vi "Compute Max Level.vi"(0 "Tone in":refnum<class "Tone.lvclass">, 1 "Filter in":refnum<class "Filter.lvclass">, 5 "Level in":refnum<class "Level.lvclass">, 7 "Fs (Hz)":dbl, 9 "Vmax":dbl, 11 "error in (no error)":errorcluster) -> (4 "Tone out":refnum<class "Tone.lvclass">, 6 "Level out":refnum<class "Level.lvclass">, 10 "Lmax":dbl, 15 "error out":errorcluster)   [LabVIEW 2020, in "Tone.lvclass"]
uses:
  Tone.lvclass
  D:/Development/epl-vi-lib/Koop/KObject Class/KObject.lvclass
  Level/Level.lvclass
  Filter/Filter.lvclass
  Tone.lvclass/Tone.ctl
  Level/Level.lvclass/Level.ctl
  82eb419d-049d-446f-8907-0d6ace39b23e.vi
  24a302fd-cf4a-4809-a84c-42078eca26b2.vi
  e33db8c1-d80d-4f9e-86c8-a606ede5ff50.vi
  937cdd26-08b4-48c4-ab2b-7b4c98fffdd3.vi
  9062d80a-ea83-4365-b942-483c8a64e32a.vi
  Level/Read Units.vi
  Koop/KObject Class/KObject.lvclass
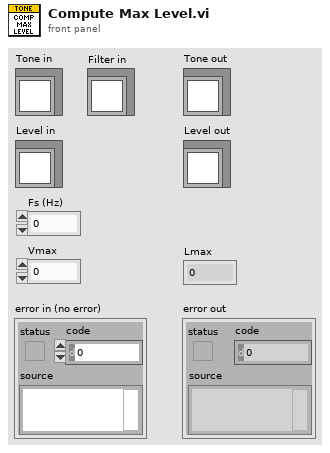
[diagram p1: front panel]
types:
  T1 = typedef "Level.lvclass/LevelUnits.ctl" = enum16{"dB atten", "dB SPL", "dB Vrms", "Volts", "dB mW", "mW", "dB HL", "dB SL"}
  T2 = cluster{"Freq (Hz)":dbl[], "Mag (dB SPL)":dbl[], "Phase (deg)":dbl[]}
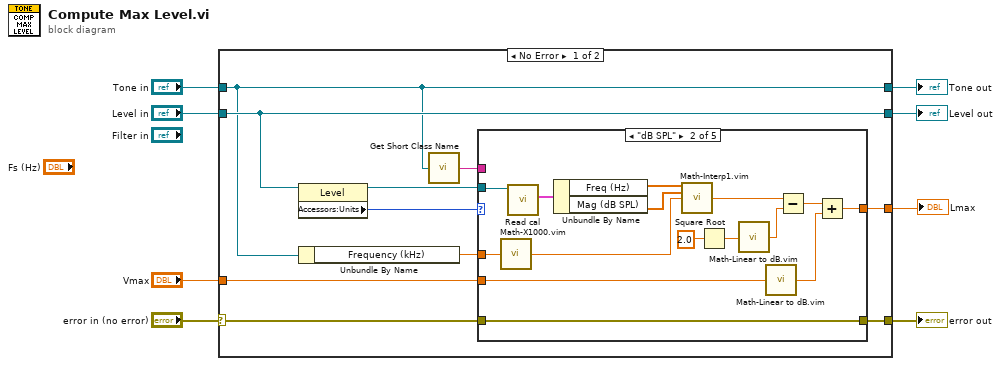
[diagram p0: block diagram]
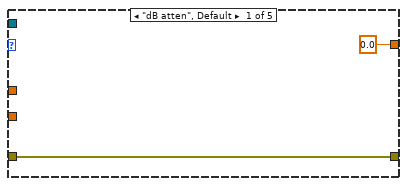
[diagram p2: hidden frame]
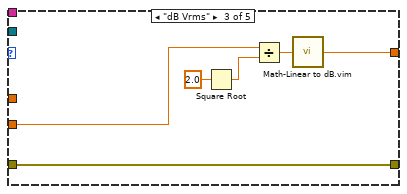
[diagram p3: hidden frame]
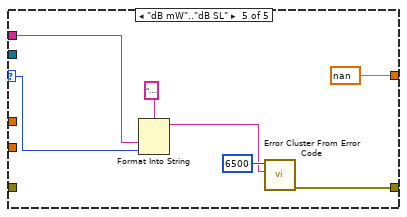
[diagram p5: hidden frame]
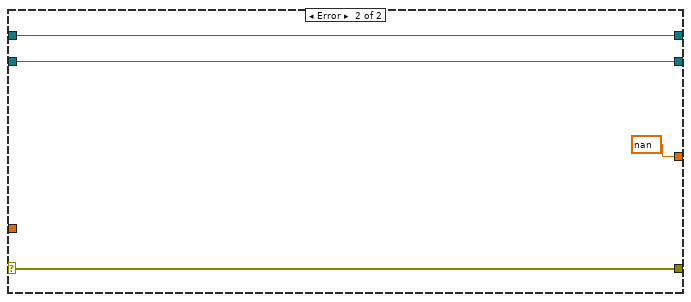
[diagram p6: hidden frame]
diagram:
  n1 = case shown="No Error" "error in (no error)" {
    selector: "error in (no error)" -> [w9 w52]
    tunnel: [w11 w54] -> w7
    tunnel: "Tone in" -> [w11 w54]
    tunnel: [w18 w53] -> w5
    tunnel: "Level in" -> [w18 w53]
    tunnel: "Vmax" -> [w13 _]
    tunnel: [w12 w52] -> w2
    tunnel: [w14 nan] -> w1
    frame No Error {
      n2 = property class="Level"(reference=w18) -> (reference out=w15:refnum<class "Level.lvclass">, "Accessors:Units"=w17:T1)  [unwired: 1 in, 1 out]
      n3 = Unbundle By Name(w11) -> ("Frequency (kHz)"=w16:dbl)
      n4 = call "Get Short Class Name.vi"("KObject in"=w11) -> ("Class"=w10:string)  [unwired: 4 in]
      n5 = case shown="\"dB SPL\"" w17 {
        selector: w17 -> [_ _ _ _ w45]
        tunnel: w16 -> [_ w35 _ _ _]
        tunnel: w15 -> [_ w24 _ _ _]
        tunnel: [0.0 w26 w37 w43 nan ("Vmax")] -> w14
        tunnel: w13 -> [_ w27 w38 w43 _]
        tunnel: [w19 w25 w36 w42 w46] -> w12
        tunnel: w10 -> [_ _ _ _ w44]
        tunnel: w9 -> [w19 w25 w36 w42 _]
        frame "dB atten", Default {
        }
        frame "dB SPL" {
          n6 = call "Math-X1000.vim"("X"=w35) -> ("1000X"=w34:dbl)
          n7 = call "Read cal.vi"("Level in"=w24) -> ("cal"=w23:T2)  [unwired: 8 in, 2 out]
          n8 = Unbundle By Name(w23) -> ("Freq (Hz)"=w22:dbl[], "Mag (dB SPL)"=w21:dbl[])
          n9 = call "Math-Interp1.vim"("X"=w22, "Y"=w21, "U"=w34) -> ("V"=w28:dbl)  [unwired: 12 in]
          n10 = Square Root(x=2.0 ("y")) -> (sqrt(x)=w31:dbl)
          n11 = call "Math-Linear to dB.vim"("linear"=w31) -> ("dB"=w32:dbl)
          n12 = call "Math-Linear to dB.vim"("linear"=w27) -> ("dB"=w29:dbl)
          n13 = Subtract(x=w28, y=w32) -> (x-y=w33:dbl)
          n14 = Add(x=w33, y=w29) -> (x+y=w26:dbl)
        }
        frame "dB Vrms" {
          n15 = Square Root(x=2.0 ("y")) -> (sqrt(x)=w40:dbl)
          n16 = Divide(x=w38, y=w40) -> (x/y=w41:dbl)
          n17 = call "Math-Linear to dB.vim"("linear"=w41) -> ("dB"=w37:dbl)
        }
        frame "Volts" {
        }
        frame "dB mW".."dB SL" {
          n18 = Format Into String(format string="%s: Cannot set level in '%s'", w44, w45) -> (resulting string=w47:string)  [unwired: 2 in, 1 out]
          n19 = call <vilib>:"Error Cluster From Error Code.vi"("error message (\"\")"=w47, "error code (0)"=6500) -> ("error out"=w46:errorcluster)  [unwired: 7 in]
        }
      }
    }
    frame Error {
    }
  }
  "error out" <- w2
  "Tone out" <- w7
  "Level out" <- w5
  "Lmax" <- w1
